vi "Get SMO HELP.vi"(8 "error in (no error)":errorcluster, 10 "Command":string, 11 "Inst.Xeryon-Rotator in":refnum<class "Inst.Xeryon-Rotator.lvclass">) -> (0 "error out":errorcluster, 2 "help cluster":T1, 3 "Inst.Xeryon-Rotator out":refnum<class "Inst.Xeryon-Rotator.lvclass">)   [LabVIEW 2019, in "Inst.Xeryon-Rotator.lvclass"]
uses:
  Inst.Xeryon-Rotator.lvclass
  <userlib>/LevyLab/Instrument Framework/Instrument/Typedefs/Instrument.IDN--cluster.ctl
  <userlib>/LevyLab/Instrument Framework/Instrument/Instrument.lvclass
  <vilib>/PRIrvin/JSON-Schema/JSON-Schema.lvlib
  <userlib>/LevyLab/Instrument Framework/Instrument Types/Cryostat/Typedefs/setAngle--cluster.ctl
  <userlib>/LevyLab/Instrument Framework/Instrument Types/Cryostat/Instrument.Cryostat.lvclass
  <userlib>/LevyLab/Instrument Framework/Instrument Types/Cryostat/Typedefs/getAngle--cluster.ctl
  Typedefs/Inst.Xeryon-Rotator.ScanState--Enum.ctl
  <userlib>/LevyLab/Instrument Framework/subsystems/Help/typedefs/Help--cluster.ctl
  <userlib>/LevyLab/Instrument Framework/subsystems/Help/Help.lvclass
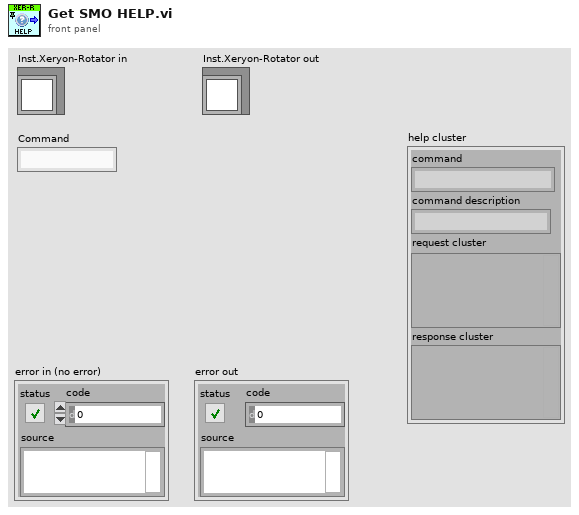
[diagram p1: front panel]
types:
  T1 = typedef "Instrument.lvlib/Help.lvclass/Help--cluster.ctl" = cluster{"command":string, "command description":string, "request cluster":variant, "response cluster":variant}
  T2 = typedef "Instrument.Cryostat.lvclass/setAngle--cluster.ctl" = cluster{"angle":dbl, "rate":dbl, "channel":i32}
  T3 = typedef "Instrument.Cryostat.lvclass/getAngle--cluster.ctl" = cluster{"angle":dbl, "status":string, "finished":bool}
  T4 = typedef "Inst.Xeryon-Rotator.lvclass/Inst.Xeryon-Rotator.ScanState--Enum.ctl" = enum16{"Scan Left", "Stop", "Scan Right"}
  T5 = typedef "Instrument.lvlib/Instrument.lvclass/Instrument.IDN--cluster.ctl" = cluster{"vendor":string, "model":string, "serial":string, "firmware":string}
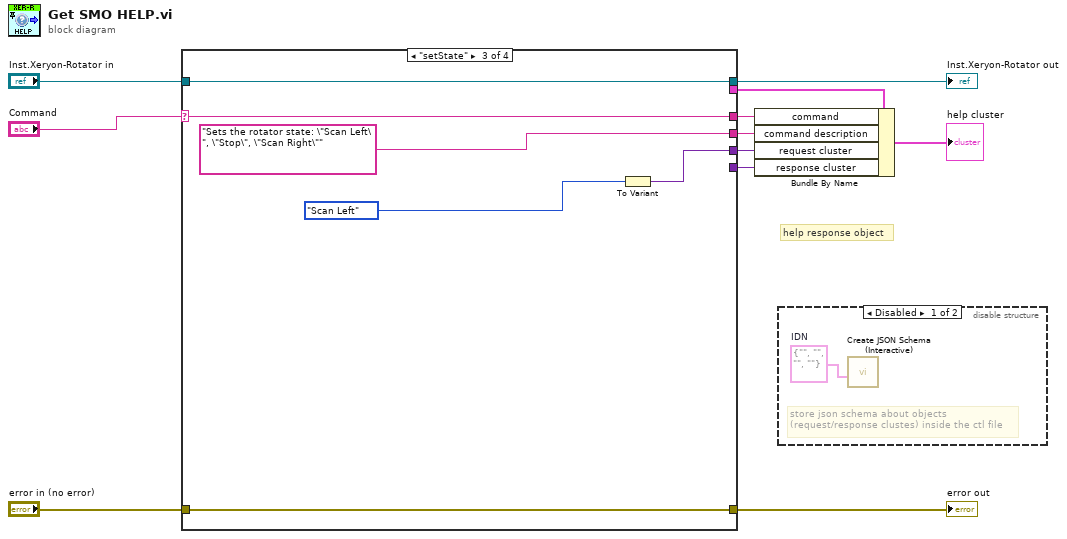
[diagram p0: block diagram]
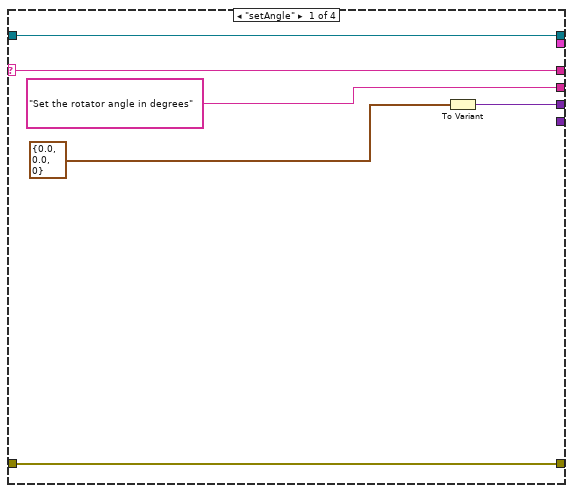
[diagram p2: hidden frame]
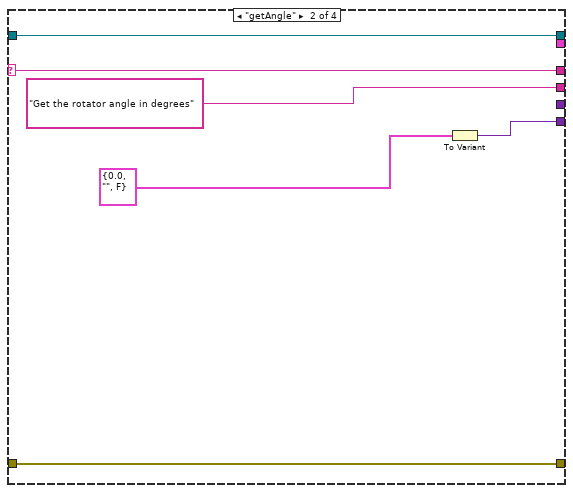
[diagram p3: hidden frame]
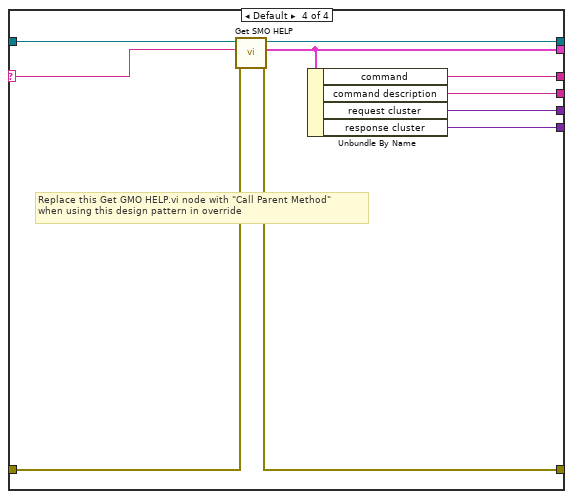
[diagram p4: hidden frame]
diagram:
  # "help response object"
  n1 = case shown="\"setState\"" "Command" {
    selector: "Command" -> [w17 w23 w29 w38]
    tunnel: [w17 w23 w29 w33] -> w5
    tunnel: "error in (no error)" -> [w16 w22 w28 w31]
    tunnel: [w16 w22 w28 w30] -> w11
    tunnel: ["Set the rotator angle in degrees" "Get the rotator angle in degrees" "Sets the rotator state: \"Scan Left\", \"Stop\", \"Scan Right\"" w34] -> w4
    tunnel: [w12 _ w24 w35] -> w3
    tunnel: [_ w18 _ w36] -> w2
    tunnel: "Inst.Xeryon-Rotator in" -> [w14 w20 w26 w39]
    tunnel: [w14 w20 w26 w37] -> w9
    tunnel: [_ _ _ w32] -> w1
    frame "setAngle" {
      n2 = To Variant(anything=T2 {"angle"=0.0, "rate"=0.0, "channel"=0} ("setAngle")) -> (Variant=w12:variant)
    }
    frame "getAngle" {
      n3 = To Variant(anything=T3 {"angle"=0.0, "status"="", "finished"=FALSE} ("getAngle")) -> (Variant=w18:variant)
    }
    frame "setState" {
      n4 = To Variant(anything=Inst.Xeryon-Rotator.ScanState--Enum."Scan Left" ("Scan State")) -> (Variant=w24:variant)
    }
    frame Default {
      # "Replace this Get GMO HELP.vi node with \"Call Parent Method\"\nwhen using this design pattern in override"
      n5 = call-parent "Get SMO HELP.vi"("error in (no error)"=w31, "Command"=w38, "Instrument in"=w39) -> ("error out"=w30:errorcluster, "help cluster"=w32:T1, "Instrument out"=w37:refnum<class "Inst.Xeryon-Rotator.lvclass">)  [unwired: 6 in]
      n6 = Unbundle By Name(w32) -> ("command"=w33:string, "command description"=w34:string, "request cluster"=w35:variant, "response cluster"=w36:variant)
    }
  }
  "Inst.Xeryon-Rotator out" <- w9
  "error out" <- w11
  n7 = Bundle By Name(cluster=w1, "command"=w5, "command description"=w4, "request cluster"=w3, "response cluster"=w2) -> (→"help cluster":T1)
  n8 = disable-structure shown="Disabled" {
    frame Disabled {
      w40 = T5 {"vendor"="", "model"="", "serial"="", "firmware"=""}  # IDN
      # "store json schema about objects\n(request/response clustes) inside the ctl file"
      n9 = call <vilib>:"Create JSON Schema (Interactive).vi"("LV Object"=w40) -> ()  [unwired: 9 in, 2 out]
    }
    frame Enabled {
    }
  }
